vi "average_all_columns_of_rand_matrix.vi"() -> ()   [LabVIEW 2021]
uses:
  <vilib>/Analysis/Matrix/Datatypes/RealMatrix.ctl
  <vilib>/Analysis/Matrix/Numeric/Conversions/Array To Matrix - RA2.vi
  <vilib>/Analysis/Matrix/NI_Matrix.lvlib
panel:
  out "avgs":dbl[](array[numeric])
  out "sink array":dbl[][](array[numeric])
  out "sink mat":T1
  out "output":dbl[][](array[numeric])
  in  "loops":dbl
  in  "blank":dbl[](array[numeric])
  out "num":dbl
  out "sum":dbl
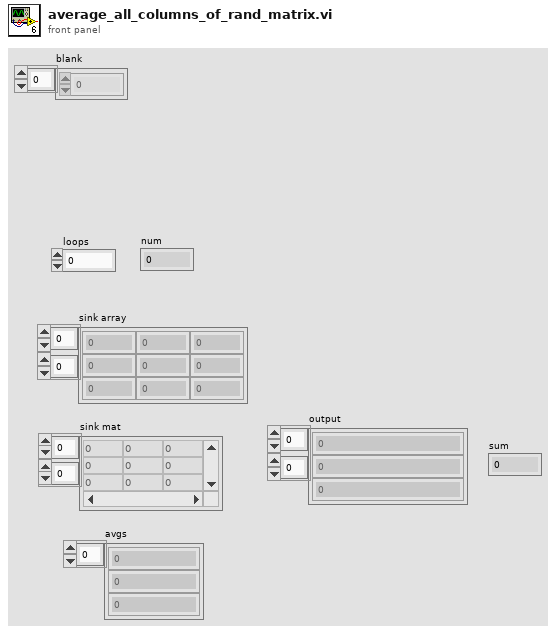
[diagram p1: front panel]
types:
  T1 = typedef "NI_Matrix.lvlib/RealMatrix.ctl" = dbl[][]
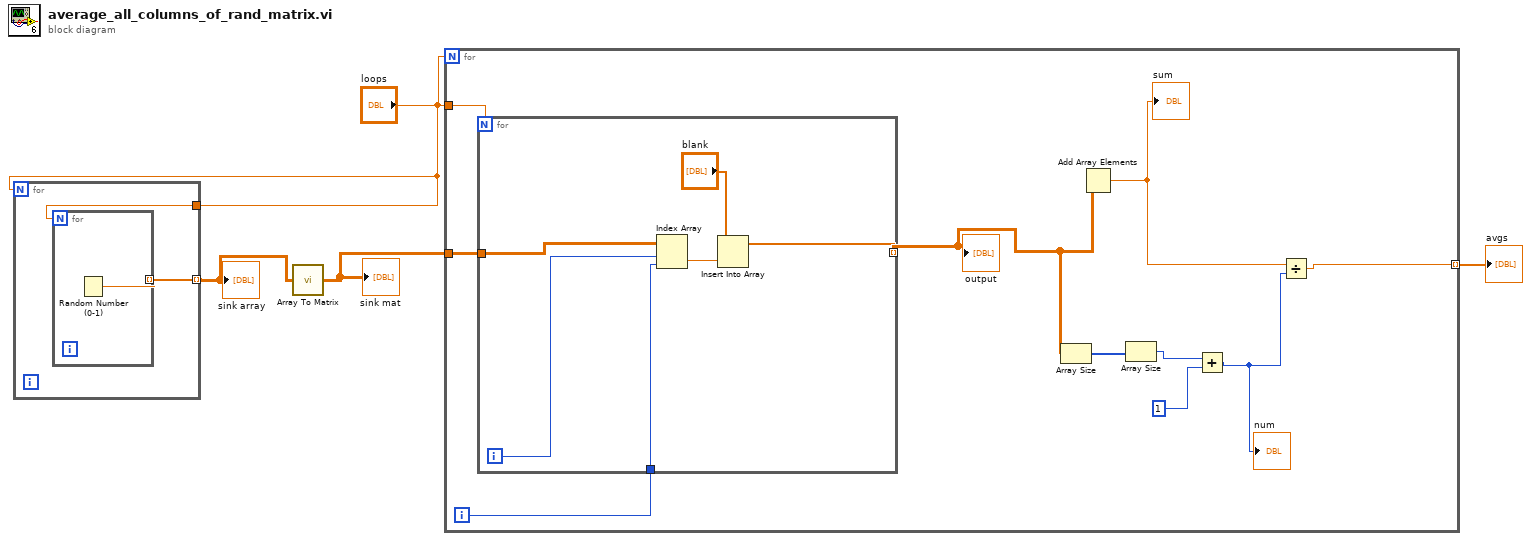
[diagram p0: block diagram]
diagram:
  n1 = for {
    N: "loops" -> [_]
    tunnel: [w6] -> w4 mode=indexing
    tunnel: "loops" -> [w5]
    n2 = for {
      N: w5 -> [_]
      tunnel: [w7] -> w6 mode=indexing
      n3 = Random Number (0-1)() -> (number: 0 to 1=w7:dbl)
    }
  }
  "sink array" <- w4
  n4 = call-poly <vilib>:"Array To Matrix.vi"("Real 2D Array"=w4) -> ("Real Matrix"=w3:T1)
  "sink mat" <- w3
  n5 = for {
    N: "loops" -> [_]
    tunnel: "loops" -> [w11]
    tunnel: w3 -> [w10]
    tunnel: [w8] -> w1 mode=indexing
    i -> [w9]
    n6 = for {
      N: w11 -> [_]
      tunnel: [w20] -> w16 mode=indexing
      tunnel: w10 -> [w19]
      tunnel: w9 -> [w18]
      i -> [w21]
      n7 = Index Array(array=w19, index (row)=w21, index (col)=w18) -> (element=w23:dbl)
      n8 = Insert Into Array(array="blank", new element=w23) -> (w20:dbl[])  [unwired: 1 in]
    }
    "output" <- w16
    n9 = Array Size(array=w16) -> (size(s)=w15:i32[])
    n10 = Add Array Elements(numeric array=w16) -> (sum=w17:dbl)
    "sum" <- w17
    n11 = Array Size(array=w15) -> (size(s)=w13:i32)
    n12 = Add(x=w13, y=1) -> (x+y=w12:i32)
    "num" <- w12
    n13 = Divide(x=w17, y=w12) -> (x/y=w8:dbl)
  }
  "avgs" <- w1
